vi "translate.vi"(0 "reference":refnum<class "AbstractNode.lvclass">, 1 "dx":dbl format="%.2f", 2 "dy":dbl format="%.2f", 5 "error in (no error)":errorcluster) -> (14 "reference out":refnum<class "AbstractNode.lvclass">, 19 "error out":errorcluster)   [LabVIEW 2016, in "AbstractNode.lvclass"]
doc: "public void translate(double dx, double dy)"
uses:
  <resource>/Framework/Providers/Open_GDS/UML/AbstractNode_class/AbstractNode.lvclass
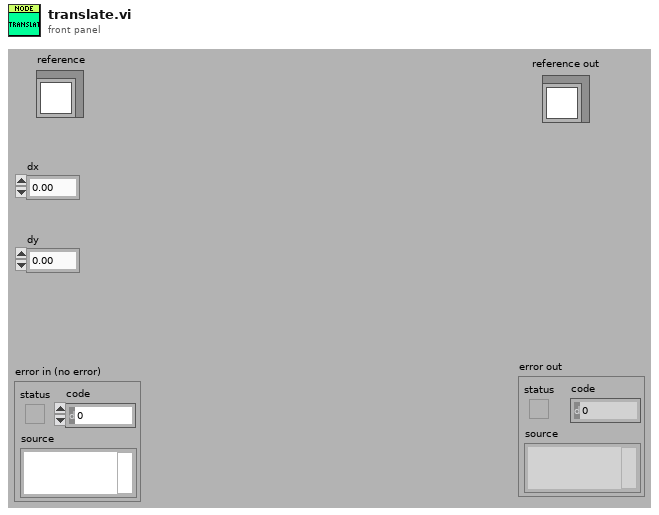
[diagram p1: front panel]
types:
  T1 = typedef "AbstractNode.lvclass/ObjectAttributes.ctl" = cluster{"parent":refnum<class "AbstractNode.lvclass">, "children":refnum<class "AbstractNode.lvclass">[], "Hidden":bool}
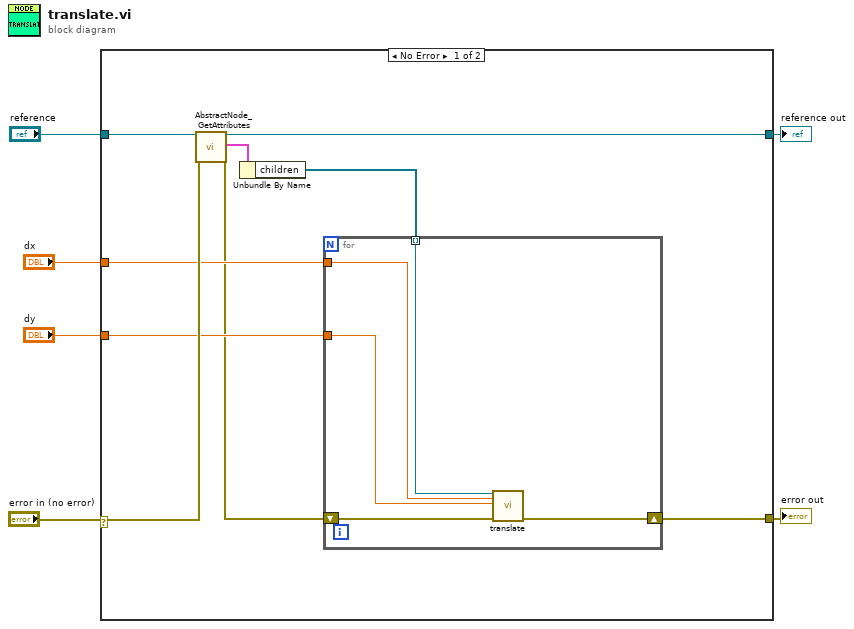
[diagram p0: block diagram]
diagram:
  n1 = case shown="No Error" "error in (no error)" {
    selector: "error in (no error)" -> [w13 w21]
    tunnel: "reference" -> [w15 w22]
    tunnel: [w8 w21] -> w5
    tunnel: [w14 w22] -> w4
    tunnel: "dx" -> [w12 _]
    tunnel: "dy" -> [w11 _]
    frame No Error {
      n2 = call <resource>:"AbstractNode_GetAttributes.vi"("reference in"=w15, "error in (no error)"=w13) -> ("reference out"=w14:refnum<class "AbstractNode.lvclass">, "Data"=w7:T1, "error out"=w9:errorcluster)  [unwired: 1 in, 14 out]
      n3 = Unbundle By Name(w7) -> ("children"=w10:refnum<class "AbstractNode.lvclass">[])
      n4 = for {
        shift-right: [w17] -> w8
        shift-left: w9 -> [w16]
        tunnel: w10 -> [w20] mode=indexing
        tunnel: w12 -> [w19]
        tunnel: w11 -> [w18]
        n5 = call-dynamic "translate.vi"("reference"=w20, "dx"=w19, "dy"=w18, "error in (no error)"=w16) -> ("error out"=w17:errorcluster)  [unwired: 14 in, 1 out]
      }
    }
    frame Error {
    }
  }
  "reference out" <- w4
  "error out" <- w5
